vi "Create New Report.vi"(8 "error in":errorcluster, 11 "Engine in":refnum<class "Engine.lvclass">) -> (0 "error out":errorcluster, 3 "Engine out":refnum<class "Engine.lvclass">)   [LabVIEW 2023, in "Engine.lvlib" / "Engine.lvclass"]
doc: "This routine enqueues a close operation followed by an open operation on the report QDMH. This guarantees that the instructions are processed in order, without interruption.\n\nThe queue consumer (report generator) is responsible for acting on the instruction set."
uses:
  Project/Engine.lvclass
  Project/Engine.lvclass/Engine.ctl
  Accessors/Read Report Queue.vi
  builds/Tools/QDMH.lvlibp/QDMH.lvclass
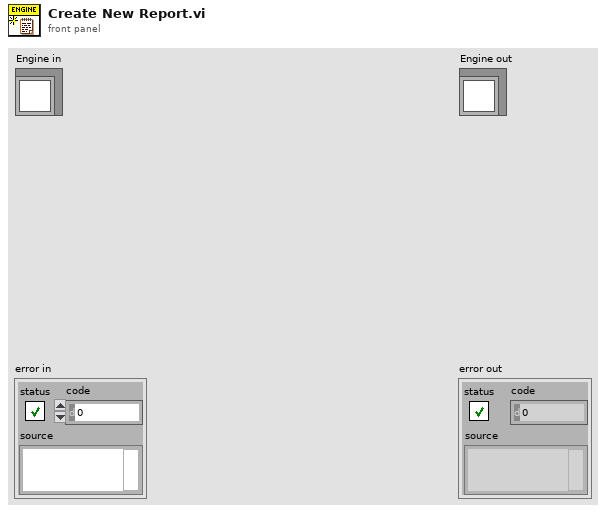
[diagram p1: front panel]
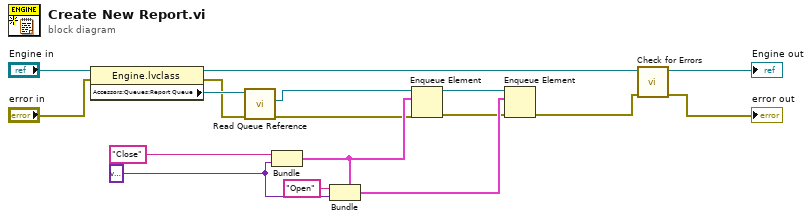
[diagram p0: block diagram]
diagram:
  w12 = variant
  n1 = property class="Engine.lvclass"(reference="Engine in", error in="error in") -> (reference out=w4:refnum<class "Engine.lvclass">, error out=w15:errorcluster, "Accessors:Queues:Report Queue"=w16:refnum<class "QDMH.lvclass">)
  n2 = call "Read Queue Reference.vi"("error in"=w15, "QDMH in"=w16) -> ("error out"=w7:errorcluster, "Queue Reference"=w8:refnum<queue>)  [unwired: 7 in, 1 out]
  n3 = Bundle("Close", w12) -> (w10:cluster{string, variant})  [unwired: 1 in]
  n4 = Bundle(cluster=w10, "Open", w12) -> (w11:cluster{string, variant})
  n5 = Enqueue Element(queue=w8, element=w10, error in (no error)=w7) -> (queue out=w5:refnum<queue>, error out=w6:errorcluster)  [unwired: 1 in, 1 out]
  n6 = Enqueue Element(queue=w5, element=w11, error in (no error)=w6) -> (error out=w2:errorcluster)  [unwired: 1 in, 2 out]
  n7 = call "Check for Errors.vi"("error in"=w2, "Engine in"=w4) -> ("error out"=→"error out":errorcluster, "Engine out"=→"Engine out":refnum<class "Engine.lvclass">)  [unwired: 8 in]
